vi "Get Register.vi"(11 "Base Attributes in":refnum<class "Base Attributes.lvclass">) -> (2 "Register":refnum<event-registration>)   [LabVIEW 2020, in "jettl.lvlib" / "Attributes.lvlib" / "Base Attributes.lvclass"]
uses:
  Base Attributes.lvclass
  Msg/Msg.lvclass
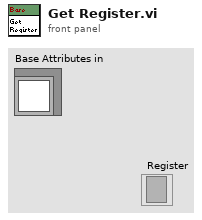
[diagram p1: front panel]
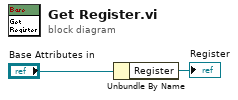
[diagram p0: block diagram]
diagram:
  n1 = Unbundle By Name("Base Attributes in") -> ("Register"=→"Register":refnum<event-registration>)
